vi "Load Hardware.vi"(8 "error in (no error)":errorcluster, 10 "Program only changes":bool=TRUE, 11 "LTA-HS in":refnum<class "LTA-HS.lvclass">) -> (0 "error out":errorcluster, 3 "LTA-HS out":refnum<class "LTA-HS.lvclass">)   [LabVIEW 2013, in "LTA-HS.lvclass"]
uses:
  LTA-HS.lvclass
  LTA-HS.lvclass/LTA-HS.ctl
  <vilib>/Utility/error.llb/DialogType.ctl
panel:
  # "encapsulate HWI in cluser so each \"last encountered\"\ncan be a different length."
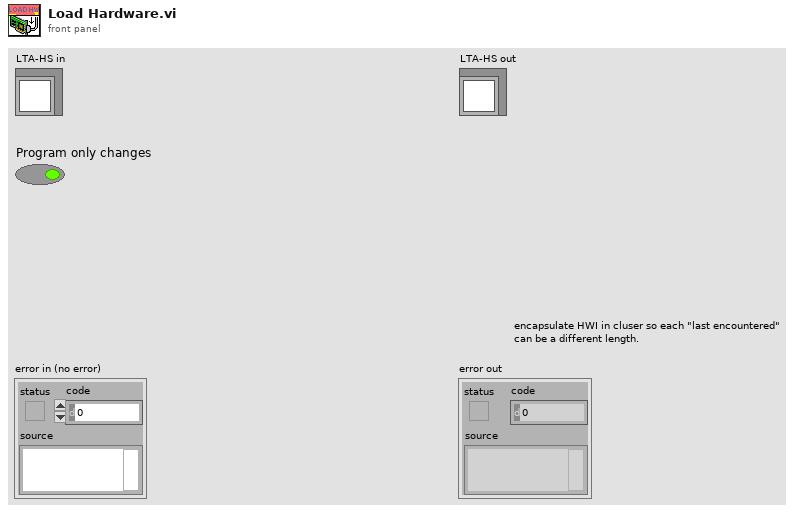
[diagram p1: front panel]
types:
  T1 = cluster{"VISA resource name":refnum<visa-resource-name>, "Device name":string, "Controller address":i32, "error":errorcluster}
  T2 = typedef "DialogType.ctl" = u16
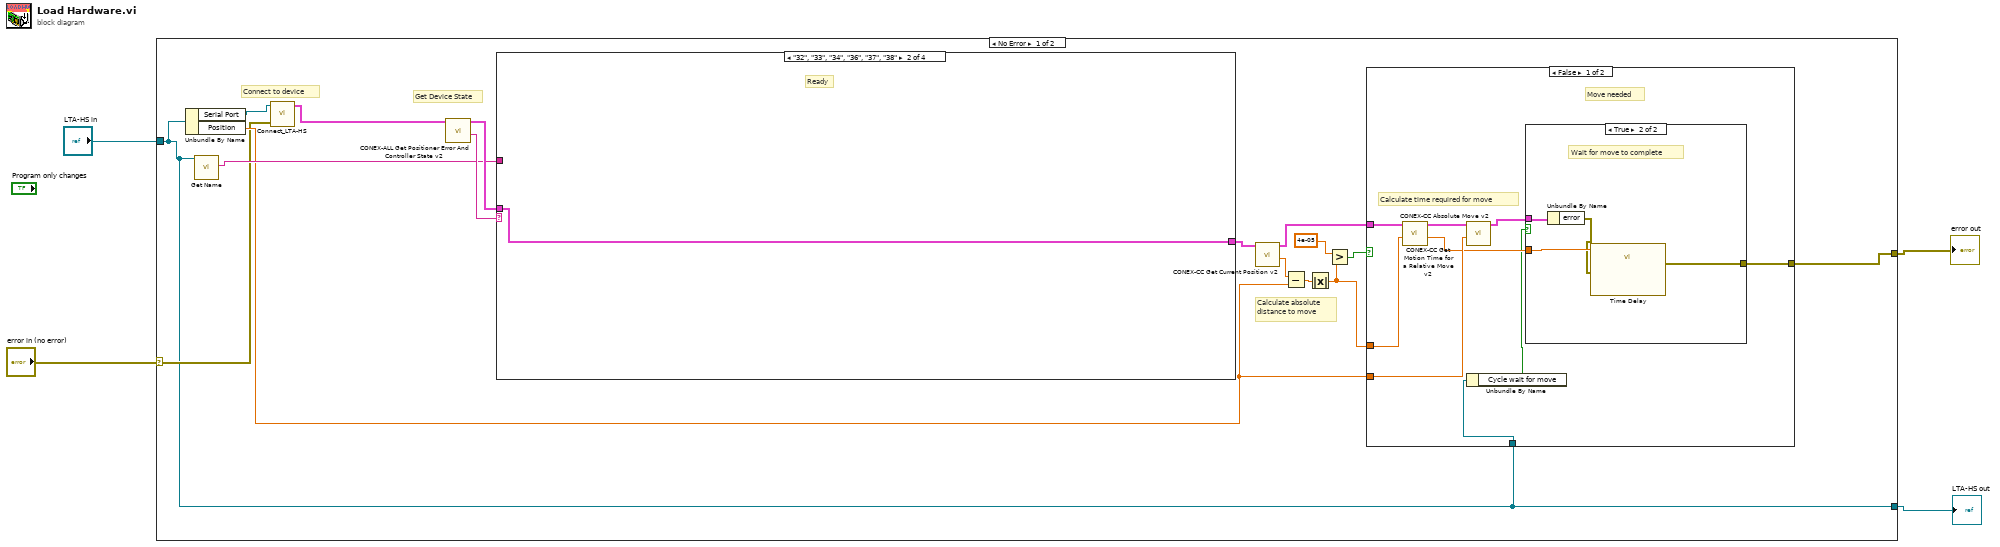
[diagram p0: block diagram]
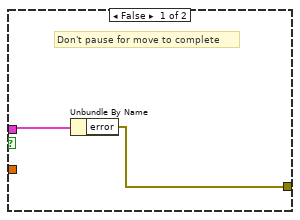
[diagram p2: hidden frame]
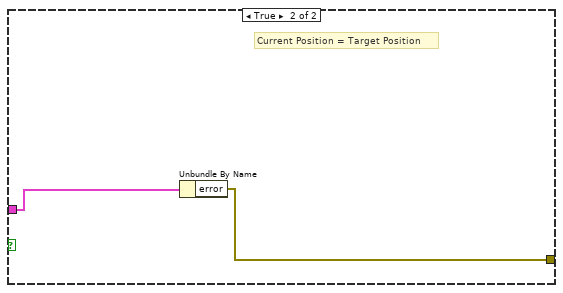
[diagram p3: hidden frame]
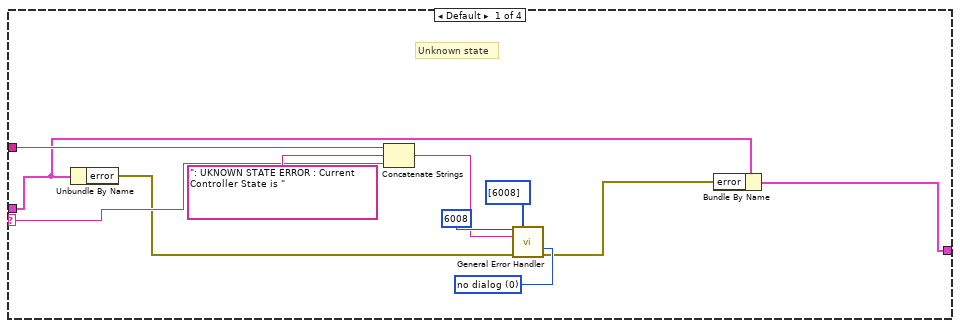
[diagram p4: hidden frame]
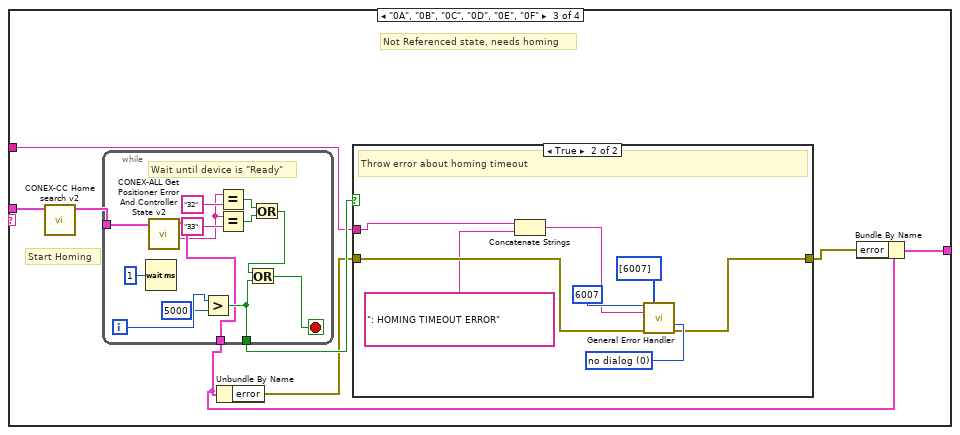
[diagram p5: hidden frame]
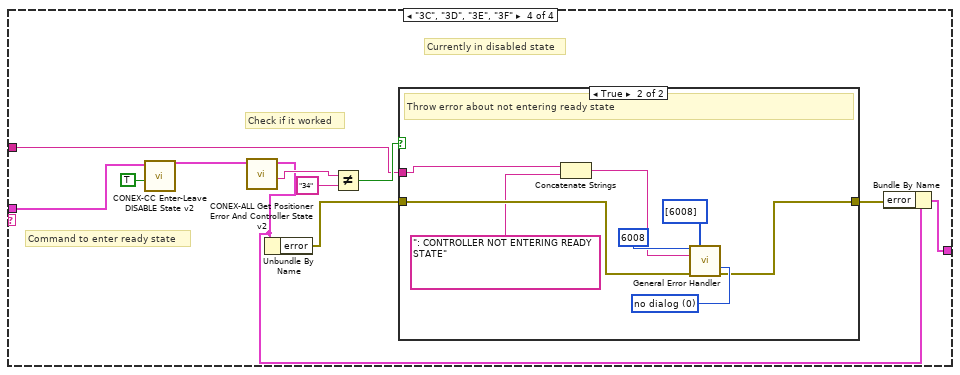
[diagram p7: hidden frame]
diagram:
  n1 = case shown="No Error" "error in (no error)" {
    selector: "error in (no error)" -> [w10 w101]
    tunnel: "LTA-HS in" -> [w5 w100]
    tunnel: [w6 w101] -> w2
    tunnel: [w5 w100] -> w1
    frame No Error {
      # "Calculate absolute \ndistance to move"
      # "Get Device State"
      # "Connect to device"
      n2 = Unbundle By Name(w5) -> ("Serial Port"=w12:refnum<visa-resource-name>, "Position"=w13:dbl)
      n3 = call-dynamic "Get Name.vi"("Device in"=w5) -> ("Name"=w18:string)  [unwired: 8 in, 2 out]
      n4 = call "Connect_LTA-HS.vi"("error in (no error)"=w10, "VISA resource name"=w12) -> ("Device Connection Cluster"=w11:T1)  [unwired: 8 in, 1 out]
      n5 = call "CONEX-ALL Get Positioner Error And Controller State v2.vi"("Connection Cluster in"=w11) -> ("Controller state"=w20:string, "Connection Cluster out"=w19:T1)  [unwired: 8 in, 1 out]
      n6 = case shown="\"32\", \"33\", \"34\", \"36\", \"37\", \"38\"" w20 {
        selector: w20 -> [w42 _ _ _]
        tunnel: w19 -> [w40 w49 w57 w90]
        tunnel: w18 -> [w43 _ w54 w84]
        tunnel: [w38 w49 w50 w80] -> w17
        frame Default {
          w48 = T2 0 items=["no dialog", "OK message", "continue or stop message", "OK message + warnings", "continue/stop + warnings"] ("type of dialog (OK msg:1)")
          # "Unknown state"
          n7 = Unbundle By Name(w40) -> ("error"=w41:errorcluster)
          n8 = Concatenate Strings(w43, ": UKNOWN STATE ERROR : Current Controller State is " ("format string"), w42) -> (w44:string)
          n9 = call <vilib>:"General Error Handler.vi"("[error code] (0)"=6008 ("error code (no error:0)"), "[user-defined codes]"=i32[] [6008], "[error source] (\" \")"=w44, "type of dialog (OK msg:1)"=w48, "error in (no error)"=w41) -> ("error out"=w39:errorcluster)  [unwired: 6 in, 4 out]
          n10 = Bundle By Name(cluster=w40, "error"=w39) -> (w38:T1)
        }
        frame "32", "33", "34", "36", "37", "38" {
          # "Ready"
        }
        frame "0A", "0B", "0C", "0D", "0E", "0F" {
          # "Start Homing"
          # "Not Referenced state, needs homing"
          n11 = call "CONEX-CC Home search v2.vi"("Connection Cluster in"=w57) -> ("Connection Cluster out"=w56:T1)  [unwired: 8 in]
          n12 = while {
            tunnel: w56 -> [w79]
            tunnel: [w69] -> w55
            tunnel: [w68] -> w52
            i -> [w71]
            stop <- w73 stop-if-true
            # "Wait until device is \"Ready\""
            n13 = Wait (ms)(milliseconds to wait=u32 1) -> ()  [unwired: 1 out]
            n14 = call "CONEX-ALL Get Positioner Error And Controller State v2.vi"("Connection Cluster in"=w79) -> ("Controller state"=w67:string, "Connection Cluster out"=w68:T1)  [unwired: 8 in, 1 out]
            n15 = Greater?(x=w71, y=5000) -> (0:w69:bool)
            n16 = Equal?(x=w67, y="32") -> (x = y?=w75:bool)
            n17 = Equal?(x=w67, y="33") -> (x = y?=w76:bool)
            n18 = Or(x=w75, y=w76) -> (x .or. y?=w74:bool)
            n19 = Or(x=w74, y=w69) -> (x .or. y?=w73:bool)
          }
          n20 = Unbundle By Name(w52) -> ("error"=w53:errorcluster)
          n21 = case shown="True" w55 {
            tunnel: w53 -> [w58 w65]
            tunnel: w54 -> [_ w61]
            tunnel: [w58 w63] -> w51
            frame False {
            }
            frame True {
              w66 = T2 0 items=["no dialog", "OK message", "continue or stop message", "OK message + warnings", "continue/stop + warnings"] ("type of dialog (OK msg:1)")
              # "Throw error about homing timeout"
              n22 = Concatenate Strings(w61, ": HOMING TIMEOUT ERROR" ("format string")) -> (w59:string)
              n23 = call <vilib>:"General Error Handler.vi"("[error code] (0)"=6007 ("error code (no error:0)"), "[user-defined codes]"=i32[] [6007], "[error source] (\" \")"=w59, "type of dialog (OK msg:1)"=w66, "error in (no error)"=w65) -> ("error out"=w63:errorcluster)  [unwired: 6 in, 4 out]
            }
          }
          n24 = Bundle By Name(cluster=w52, "error"=w51) -> (w50:T1)
        }
        frame "3C", "3D", "3E", "3F" {
          # "Check if it worked"
          # "Command to enter ready state"
          # "Currently in disabled state"
          n25 = call "CONEX-CC Enter-Leave DISABLE State v2.vi"("Ready? (false=DISABLE true=READY)"=TRUE, "Connection Cluster in"=w90) -> ("Connection Cluster out"=w88:T1)  [unwired: 7 in]
          n26 = call "CONEX-ALL Get Positioner Error And Controller State v2.vi"("Connection Cluster in"=w88) -> ("Controller state"=w86:string, "Connection Cluster out"=w82:T1)  [unwired: 8 in, 1 out]
          n27 = Unbundle By Name(w82) -> ("error"=w83:errorcluster)
          n28 = Not Equal?(x=w86, y="34") -> (x != y?=w85:bool)
          n29 = case shown="True" w85 {
            tunnel: w83 -> [w91 w98]
            tunnel: w84 -> [_ w94]
            tunnel: [w91 w96] -> w81
            frame False {
            }
            frame True {
              w99 = T2 0 items=["no dialog", "OK message", "continue or stop message", "OK message + warnings", "continue/stop + warnings"] ("type of dialog (OK msg:1)")
              # "Throw error about not entering ready state"
              n30 = Concatenate Strings(w94, ": CONTROLLER NOT ENTERING READY STATE" ("format string")) -> (w92:string)
              n31 = call <vilib>:"General Error Handler.vi"("[error code] (0)"=6008 ("error code (no error:0)"), "[user-defined codes]"=i32[] [6008], "[error source] (\" \")"=w92, "type of dialog (OK msg:1)"=w99, "error in (no error)"=w98) -> ("error out"=w96:errorcluster)  [unwired: 6 in, 4 out]
            }
          }
          n32 = Bundle By Name(cluster=w82, "error"=w81) -> (w80:T1)
        }
      }
      n33 = call "CONEX-CC Get Current Position v2.vi"("Connection Cluster in"=w17) -> ("Current position"=w15:dbl, "Connection Cluster out"=w16:T1)  [unwired: 8 in, 1 out]
      n34 = Subtract(x=w15, y=w13) -> (x-y=w14:dbl)
      n35 = Absolute Value(x=w14) -> (abs(x)=w8:dbl)
      n36 = Greater?(x=4e-05, y=w8) -> (0:w7:bool)
      n37 = case shown="False" w7 {
        tunnel: w16 -> [w29 w37]
        tunnel: w8 -> [w28 _]
        tunnel: w13 -> [w26 _]
        tunnel: w5 -> [w23 _]
        tunnel: [w21 w36] -> w6
        frame False {
          # "Calculate time required for move"
          # "Move needed"
          n38 = call "CONEX-CC Get Motion Time for a Relative Move v2.vi"("Displacement"=w28, "Connection Cluster in"=w29) -> ("Motion Time (s)"=w25:dbl, "Connection Cluster out"=w27:T1)  [unwired: 7 in, 1 out]
          n39 = call "CONEX-CC Absolute Move v2.vi"("Target position"=w26, "Connection Cluster in"=w27) -> ("Connection Cluster out"=w24:T1)  [unwired: 7 in]
          n40 = Unbundle By Name(w23) -> ("Cycle wait for move"=w22:bool)
          n41 = case shown="True" w22 {
            tunnel: w25 -> [_ w35]
            tunnel: w24 -> [w31 w33]
            tunnel: [w30 w32] -> w21
            frame False {
              # "Don't pause for move to complete"
              n42 = Unbundle By Name(w31) -> ("error"=w30:errorcluster)
            }
            frame True {
              # "Wait for move to complete"
              n43 = Unbundle By Name(w33) -> ("error"=w34:errorcluster)
              n44 = call "Time Delay"("error in (no error)"=w34, "Delay Time (s)"=w35) -> ("error out"=w32:errorcluster)  [unwired: 9 in]
            }
          }
        }
        frame True {
          # "Current Position = Target Position"
          n45 = Unbundle By Name(w37) -> ("error"=w36:errorcluster)
        }
      }
    }
    frame Error {
    }
  }
  "error out" <- w2
  "LTA-HS out" <- w1
